vi "Read Accelerometer.vi"(8 "error in (no error)":errorcluster, 10 "accel range (m/s2)":dbl=2.0, 11 "Accelerometer":T1) -> (0 "error out":errorcluster, 2 "data":dbl[](array[numeric]), 3 "Accelerometer out":T1)   [LabVIEW 2012]
doc: "Use this template to build a VI to use as a subVI."
uses:
  Accelerometer.ctl
  <vilib>/ni845x/ni845x.llb/ni845xControl.ctl
  <vilib>/ni845x/ni845x.llb/ni845xI2cConfiguration.ctl
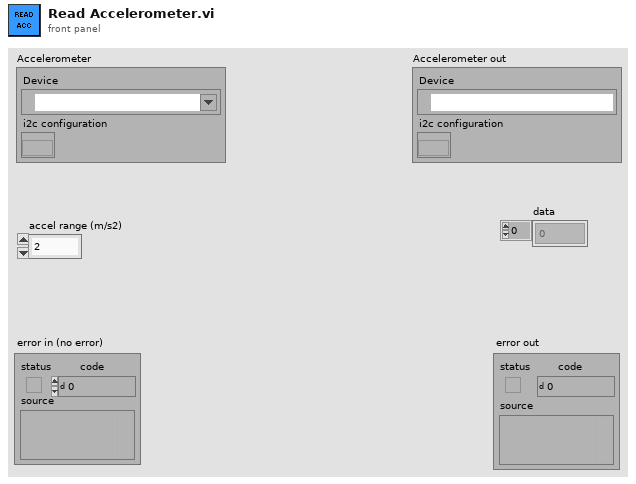
[diagram p1: front panel]
types:
  T1 = typedef "Accelerometer.ctl" = cluster{"Device":T2, "i2c configuration":T3}
  T2 = typedef "ni845xControl.ctl" = refnum<k21>
  T3 = typedef "ni845xI2cConfiguration.ctl" = refnum<k20>
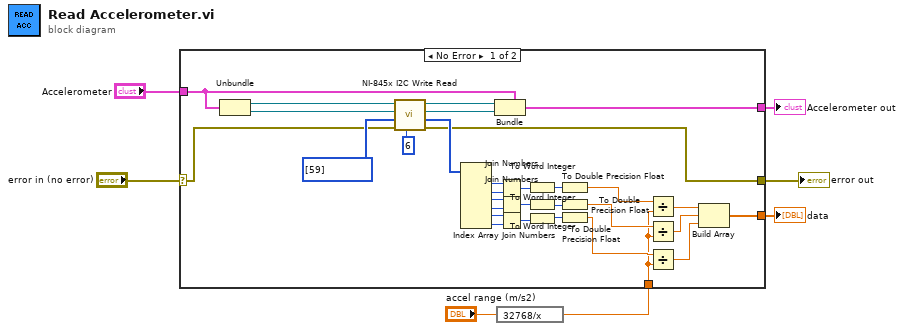
[diagram p0: block diagram]
diagram:
  n1 = expression code="32768/x"("accel range (m/s2)") -> (w2:dbl)
  n2 = case shown="No Error" "error in (no error)" {
    selector: "error in (no error)" -> [w9 w40]
    tunnel: [w8 w40] -> w6
    tunnel: "Accelerometer" -> [w32 w39]
    tunnel: [w31 w39] -> w4
    tunnel: w2 -> [w14 _]
    tunnel: [w10 _] -> w1
    frame No Error {
      n3 = Unbundle(w32) -> ("Device"=w36:T2, "i2c configuration"=w35:T3)
      n4 = call <vilib>:"NI-845x I2C Write Read.vi"("num bytes to read"=u32 6, "error in (no error)"=w9, "write data"=u8[] [59], "i2c configuration in"=w35, "device reference in"=w36) -> ("error out"=w8:errorcluster, "read data"=w30:u8[], "i2c configuration out"=w33:T3, "device reference out"=w34:T2)  [unwired: 3 in]
      n5 = Index Array(array=w30) -> (element #1=w28:u8, element #2=w29:u8, element #3=w25:u8, element #4=w27:u8, element #5=w24:u8, element #6=w26:u8)  [unwired: 6 in]
      n6 = Bundle(cluster=w32, "Device"=w34, "i2c configuration"=w33) -> (w31:T1)
      n7 = Join Numbers(hi=w28, lo=w29) -> ((hi.lo)=w17:u16)
      n8 = Join Numbers(hi=w25, lo=w27) -> ((hi.lo)=w16:u16)
      n9 = Join Numbers(hi=w24, lo=w26) -> ((hi.lo)=w15:u16)
      n10 = To Word Integer(number=w17) -> (16bit integer=w18:i16)
      n11 = To Word Integer(number=w16) -> (16bit integer=w19:i16)
      n12 = To Word Integer(number=w15) -> (16bit integer=w20:i16)
      n13 = To Double Precision Float(number=w18) -> (double precision float=w21:dbl)
      n14 = To Double Precision Float(number=w19) -> (double precision float=w22:dbl)
      n15 = To Double Precision Float(number=w20) -> (double precision float=w23:dbl)
      n16 = Divide(x=w21, y=w14) -> (x/y=w13:dbl)
      n17 = Divide(x=w22, y=w14) -> (x/y=w12:dbl)
      n18 = Divide(x=w23, y=w14) -> (x/y=w11:dbl)
      n19 = Build Array(w13, w12, w11) -> (w10:dbl[])
    }
    frame Error {
    }
  }
  "error out" <- w6
  "Accelerometer out" <- w4
  "data" <- w1
